vi "Get Type Details.vi"(8 "error in (no error)":errorcluster, 10 "Name":string, 11 "IoT Session in":refnum<class "IoT Session.lvclass">) -> (0 "error out":errorcluster, 2 "Details":T1, 3 "IoT Session out":refnum<class "IoT Session.lvclass">)   [LabVIEW 2015, in "NI_AWS_IoT.lvlib" / "IoT Session.lvclass"]
uses:
  IoT Session.lvclass
  Type.ctl
  Core/HTTP Request/Request Options.ctl
  Core/HTTP Request/Name Value Pair.ctl
  Core/HTTP Request/Region handling.ctl
  Core/HTTP Request/URL formatting.ctl
  Core/HTTP Request/HTTP Request.lvclass
  NI_AWS_IoT.lvlib
  JSON Parsing/NI_JSON Parsing.lvlib
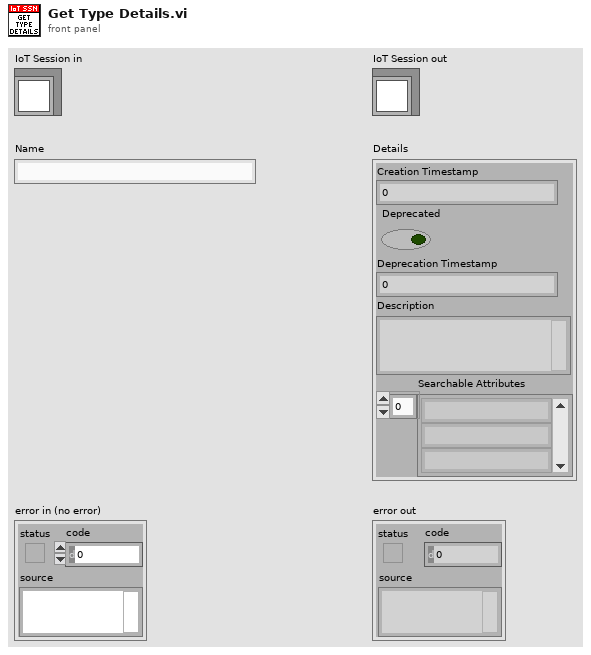
[diagram p1: front panel]
types:
  T1 = typedef "NI_AWS_IoT.lvlib/Type.ctl" = cluster{"Creation Timestamp":dbl, "Deprecated":bool, "Deprecation Timestamp":dbl, "Description":string, "Searchable Attributes":string[]}
  T2 = typedef "NI_AWS_Core.lvlib/HTTP Request.lvclass/Name Value Pair.ctl" = cluster{"name":string, "value":string}
  T3 = typedef "NI_AWS_Core.lvlib/HTTP Request.lvclass/Request Options.ctl" = cluster{"request headers":T2[], "request parameters":T2[], "request body":string, "region handling":T4, "URL formatting":T5}
  T4 = typedef "NI_AWS_Core.lvlib/HTTP Request.lvclass/Region handling.ctl" = enum16{"use region everywhere", "use region (authentication only)", "use region (URL only)", "ignore region everwhere"}
  T5 = typedef "NI_AWS_Core.lvlib/HTTP Request.lvclass/URL formatting.ctl" = enum16{"region-", "region."}
  T6 = typedef "NI_AWS_Core.lvlib/HTTP Request.lvclass/Response.ctl" = cluster{"Headers":string, "Body":string}
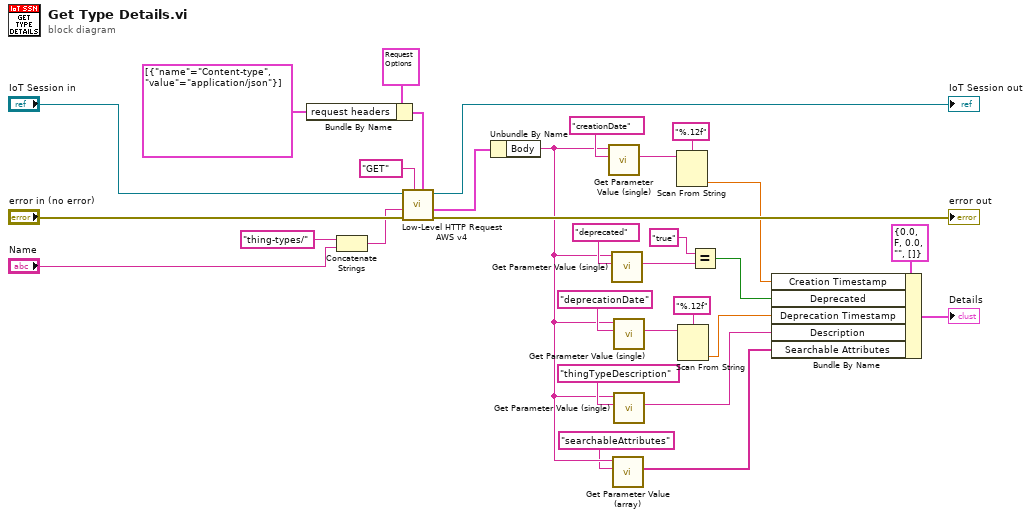
[diagram p0: block diagram]
diagram:
  n1 = Bundle By Name(cluster=T3 {"request headers"=[], "request parameters"=[], "request body"="", "region handling"=enum."use region everywhere", "URL formatting"=enum."region."} ("Request Options"), "request headers"=T2[] [{"name"="Content-type", "value"="application/json"}]) -> (w25:T3)
  n2 = Concatenate Strings("thing-types/" ("string"), "Name") -> (w21:string)
  n3 = call "Low-Level HTTP Request AWS v4.vi"("Request Options"=w25, "HTTP-Verb"="GET", "error in (no error)"="error in (no error)", "URL Suffix"=w21, "AWS Core in"="IoT Session in") -> ("error out"=→"error out":errorcluster, "Response"=w23:T6, "AWS Core out"=→"IoT Session out":refnum<class "IoT Session.lvclass">)  [unwired: 3 in, 1 out]
  n4 = Unbundle By Name(w23) -> ("Body"=w10:string)
  n5 = call "Get Parameter Value (single).vi"("Parameter Name"="creationDate", "JSON"=w10) -> ("Parameter Value"=w6:string)  [unwired: 6 in, 3 out]
  n6 = call "Get Parameter Value (single).vi"("Parameter Name"="deprecated", "JSON"=w10) -> ("Parameter Value"=w1:string)  [unwired: 6 in, 3 out]
  n7 = call "Get Parameter Value (array).vi"("Parameter Name"="searchableAttributes", "JSON"=w10) -> ("Parameter Values"=w8:string[])  [unwired: 7 in, 2 out]
  n8 = call "Get Parameter Value (single).vi"("Parameter Name"="deprecationDate", "JSON"=w10) -> ("Parameter Value"=w3:string)  [unwired: 6 in, 3 out]
  n9 = call "Get Parameter Value (single).vi"("Parameter Name"="thingTypeDescription", "JSON"=w10) -> ("Parameter Value"=w11:string)  [unwired: 6 in, 3 out]
  n10 = Scan From String(format string="%.12f", input string=w6) -> (output 1=w5:dbl)  [unwired: 3 in, 3 out]
  n11 = Scan From String(format string="%.12f", input string=w3) -> (output 1=w2:dbl)  [unwired: 3 in, 3 out]
  n12 = Equal?(x="true", y=w1) -> (x = y?=w13:bool)
  n13 = Bundle By Name(cluster=T1 {"Creation Timestamp"=0.0, "Deprecated"=FALSE, "Deprecation Timestamp"=0.0, "Description"="", "Searchable Attributes"=[]} ("Details"), "Creation Timestamp"=w5, "Deprecated"=w13, "Deprecation Timestamp"=w2, "Description"=w11, "Searchable Attributes"=w8) -> (→"Details":T1)
